vi "Edit Thirukkural File.vi"() -> ()   [LabVIEW 2019]
uses:
  <userlib>/APTLib.lnk/File IO/_Read Write Data File _APTLib.llb/File IO Option _APTLib.ctl
  <userlib>/APTLib.lnk/File IO/_Read Write Data File _APTLib.llb/Text Encoding Format _APTLib.ctl
  <userlib>/APTLib.lnk/File IO/_Read Write Data File _APTLib.llb/Read Write Unicode Text File _APTLib.vi
panel:
  out "Numeric":i32
  out "error out":errorcluster
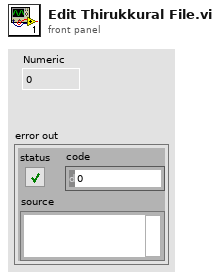
[diagram p1: front panel]
types:
  T1 = typedef "Text Encoding Format _APTLib.ctl" = enum8{"ASCII", "UTF-8", "UTF-16 LE", "UTF-16 BE"}
  T2 = typedef "File IO Option _APTLib.ctl" = enum16{"Read", "Write"}
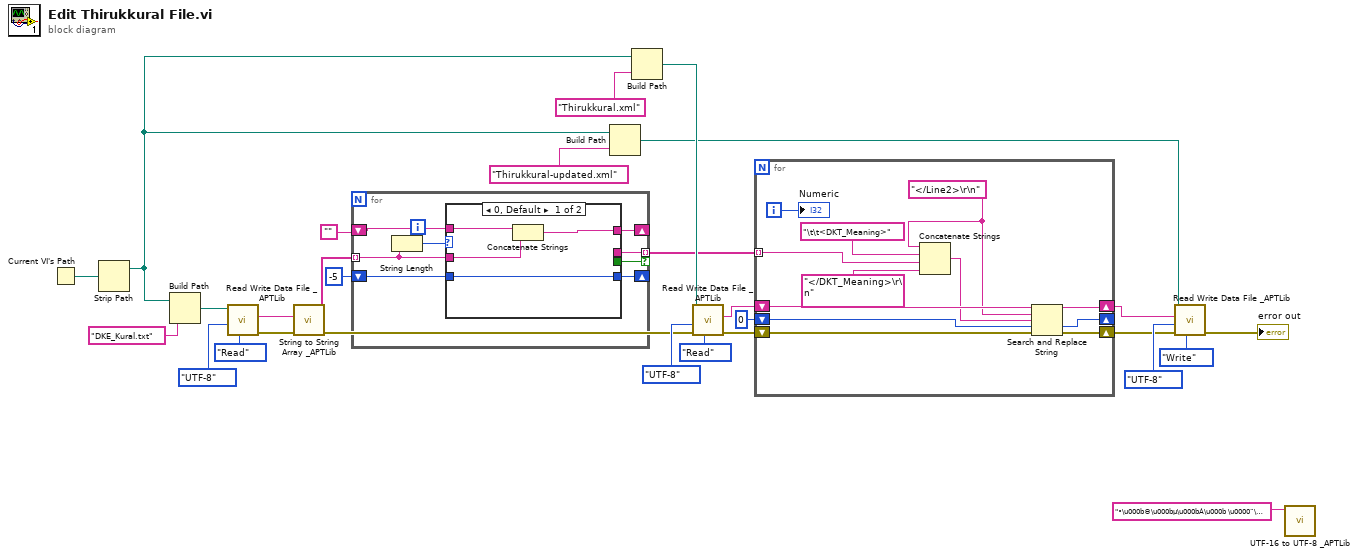
[diagram p0: block diagram]
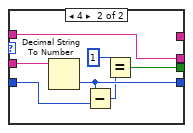
[diagram p2: hidden frame]
diagram:
  n1 = Current VI's Path() -> (path=w22:path)
  n2 = Strip Path(path=w22) -> (stripped path=w11:path)  [unwired: 1 out]
  n3 = Build Path(base path=w11, name or relative path="DKE_Kural.txt") -> (appended path=w27:path)
  n4 = call-poly <userlib>:"Read Write Data File _APTLib.vi"("Option"=File_IO_Option__APTLib."Read", "Encoding?"=Text_Encoding_Format__APTLib."UTF-8", "file path"=w27) -> ("error out"=w19:errorcluster, "String Out"=w20:string)  [unwired: 6 in, 1 out]
  n5 = call <userlib>:"String to String Array _APTLib.vi"("error in"=w19, "String Input"=w20) -> ("error out"=w18:errorcluster, "String Array"=w4:string[])  [unwired: 8 in]
  n6 = for {
    tunnel: w4 -> [w34] mode=indexing
    tunnel: [w36] -> w3 mode=indexing if=w29
    shift-right: [w33] -> _
    shift-left: -5 -> [w32]
    shift-right: [w30] -> _
    shift-left: "" -> [w31]
    n7 = String Length(string=w34) -> (length=w35:i32)
    n8 = case shown="0, Default" w35 {
      tunnel: [_ w41] -> w36
      tunnel: w34 -> [w38 w47]
      tunnel: [w40 w46] -> w33
      tunnel: w32 -> [w40 w45]
      tunnel: [_ w42] -> w29
      tunnel: w31 -> [w39 w41]
      tunnel: [w37 _] -> w30
      frame 0, Default {
        n9 = Concatenate Strings(w39, w38) -> (w37:string)
      }
      frame 4 {
        n10 = Decimal String To Number(string=w47) -> (number=w46:i32)  [unwired: 2 in, 1 out]
        n11 = Subtract(x=w46, y=w45) -> (x-y=w44:i32)
        n12 = Equal?(x=1 ("y"), y=w44) -> (x = y?=w42:bool)
      }
    }
  }
  n13 = Build Path(base path=w11, name or relative path="Thirukkural-updated.xml") -> (appended path=w8:path)
  n14 = Build Path(base path=w11, name or relative path="Thirukkural.xml") -> (appended path=w24:path)
  n15 = call-poly <userlib>:"Read Write Data File _APTLib.vi"("Option"=File_IO_Option__APTLib."Read", "error in"=w18, "Encoding?"=Text_Encoding_Format__APTLib."UTF-8", "file path"=w24) -> ("error out"=w17:errorcluster, "String Out"=w16:string)  [unwired: 5 in, 1 out]
  n16 = for {
    shift-right: [w59] -> w13
    shift-left: w17 -> [w58]
    tunnel: w3 -> [w56] mode=indexing
    shift-right: [w51] -> w7
    shift-left: w16 -> [w54]
    shift-right: [w53] -> _
    shift-left: 0 ("offset past replacement") -> [w52]
    i -> [w48]
    w50 = "</Line2>\r\n" ("search string")
    n17 = Concatenate Strings(w50, "\t\t<DKT_Meaning>", w56, "</DKT_Meaning>\r\n") -> (w49:string)
    n18 = Search and Replace String(input string=w54, search string=w50, replace string=w49, offset=w52, error in=w58) -> (result string=w51:string, offset past replacement=w53:i32, error out=w59:errorcluster)  [unwired: 3 in, 1 out]
    "Numeric" <- w48
  }
  n19 = call-poly <userlib>:"Read Write Data File _APTLib.vi"("Option"=File_IO_Option__APTLib."Write", "error in"=w13, "Encoding?"=Text_Encoding_Format__APTLib."UTF-8", "String In"=w7, "file path"=w8) -> ("error out"=→"error out":errorcluster)  [unwired: 4 in, 2 out]
  n20 = call <userlib>:"UTF-16 to UTF-8 _APTLib.vi"("UTF-16 String"="•\u000b©\u000bµ\u000bÁ\u000b \u0000¨\u000b¿\u000b²\u000bÈ\u000b \u0000‰\u000b°\u000bÈ\u000b¤\u000bÍ\u000b¤\u000b²\u000bÍ\u000b" ("String")) -> ()  [unwired: 9 in, 2 out]
